vi "例4.11-2 循环结构.vi"() -> ()   [LabVIEW 2017]
panel:
  out "数组":i32[](array[numeric])
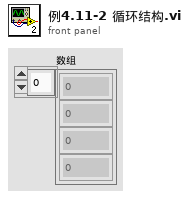
[diagram p1: front panel]
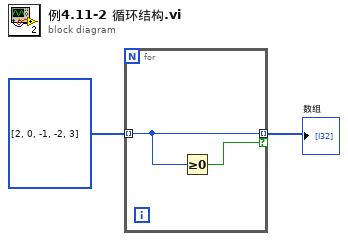
[diagram p0: block diagram]
diagram:
  n1 = for {
    tunnel: i32[] [2, 0, -1, -2, 3] -> [w4] mode=indexing
    tunnel: [w4] -> w2 mode=indexing if=w3
    n2 = Greater Or Equal To 0?(x=w4) -> (x >= 0?=w3:bool)
  }
  "数组" <- w2
